vi "ECG.vi"() -> ()   [LabVIEW 2016]
uses:
  <vilib>/Analysis/3filter.llb/Filter Passband Type.ctl
  <vilib>/ptbypt/NI_PtbyPt.lvlib
  <vilib>/Analysis/NI_AALBase.lvlib
panel:
  in  "stop 2":bool
  in  "stop":bool
  in  "submit":bool
  out "Prompt":string="Update or Confirm the Following Information:"
  out "Pat":string="Patient Name:"
  out "Dat":string="Date/Time:"
  out "time string 2":string
  out "date string 2":string
  in  "Name 2":string="Doe, John"
  in  "Notes:":string
  out "Box":string
  in  "Notes:":string
  out "String":string
  out "Elapsed Time (s)":dbl format="%<%H:%M:%S>t"
  out "time string":string
  out "date string":string
  out "Heart":bool
  in  "Name":string="Doe, John"
  in  "T Thresh":string="100"
  in  "B Thresh":string="60"
  out "Bradycardia":bool
  out "Tachycardia":bool
  out "HR":dbl=56.0
  out "String 2":string
  out "Waveform Chart":dbl(graph)
  # "Patient Name:"
  # "Date/Time:"
  # "HR"
  # "bpm"
  # "Set Thresholds:"
  # "Bradycardia"
  # "Tachycardia"
  # "Time Elapsed:"
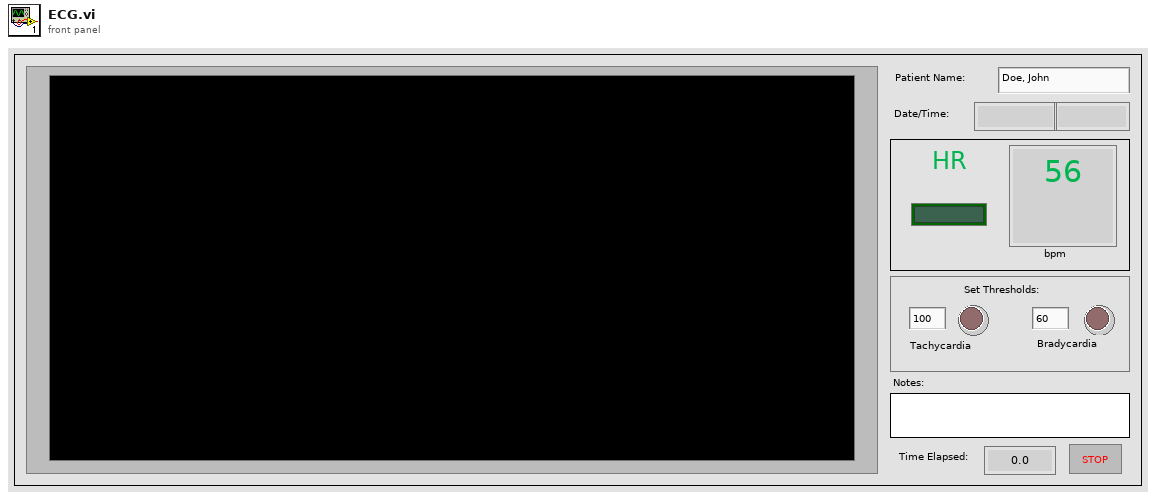
[diagram p1: front panel]
types:
  T1 = typedef "NI_AALBase.lvlib/Filter Passband Type.ctl" = enum32{"Lowpass", "Highpass", "Bandpass", "Bandstop"}
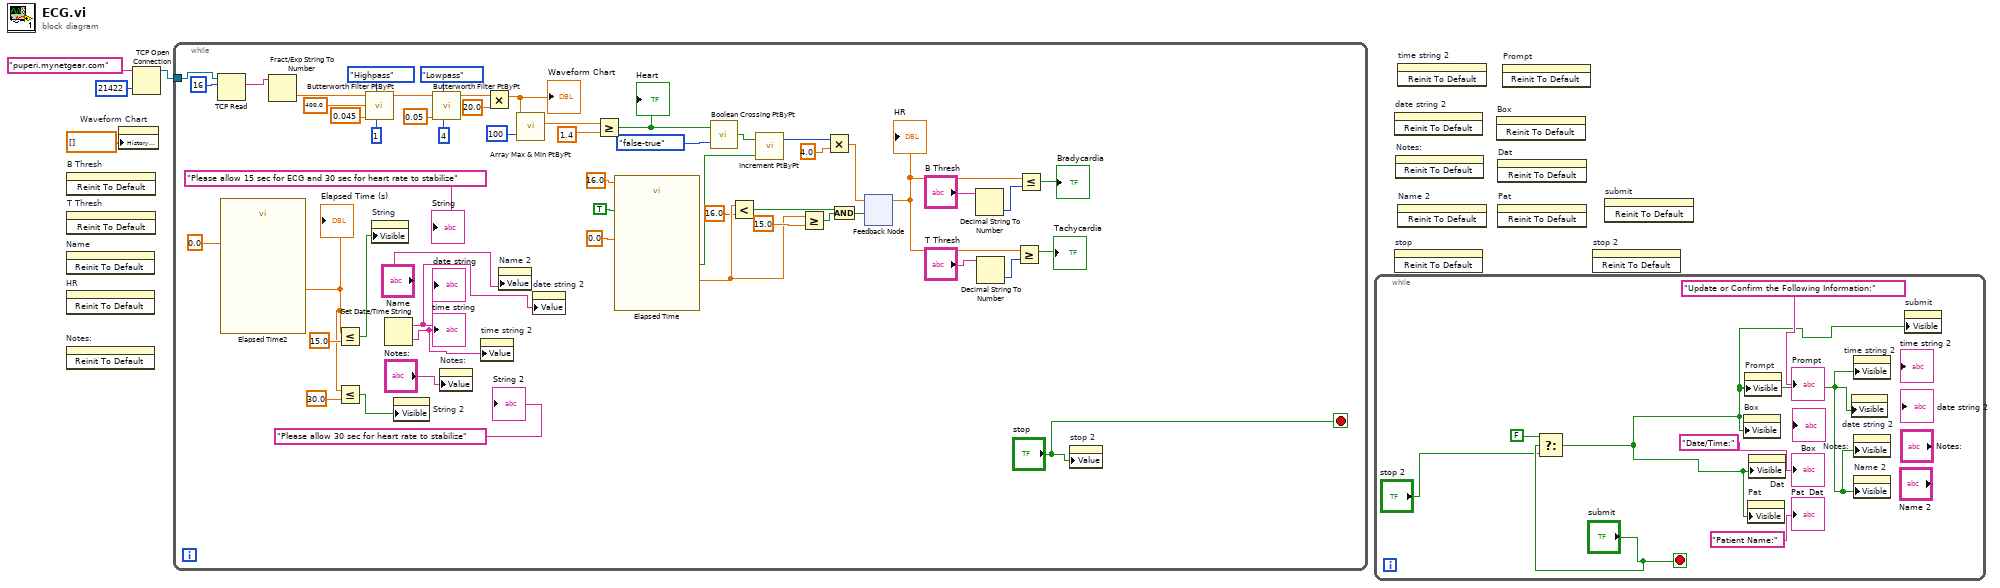
[diagram p0: block diagram]
diagram:
  n1 = invoke on="Name" class="Str" method="Reinit To Default"() -> ()  [unwired: 3 in, 3 out]
  n2 = invoke on="HR" class="DigNum (strict)" method="Reinit To Default"() -> ()  [unwired: 3 in, 3 out]
  n3 = invoke on="Notes:" class="Str" method="Reinit To Default"() -> ()  [unwired: 3 in, 3 out]
  n4 = invoke on="B Thresh" class="Str" method="Reinit To Default"() -> ()  [unwired: 3 in, 3 out]
  n5 = invoke on="T Thresh" class="Str" method="Reinit To Default"() -> ()  [unwired: 3 in, 3 out]
  n6 = property on="Waveform Chart" class="WFChart (strict)"("History Data"=dbl[] []) -> ()  [unwired: 2 in, 2 out]
  n7 = TCP Open Connection(address="puperi.mynetgear.com", remote port or service name=u16 21422) -> (connection ID=w2:refnum<k5>)  [unwired: 3 in, 1 out]
  n8 = while {
    tunnel: w2 -> [w58]
    stop <- "stop" stop-if-true
    n9 = TCP Read(connection ID=w58, bytes to read=16) -> (data out=w51:string)  [unwired: 3 in, 2 out]
    n10 = call "Elapsed Time2"("Set Start Time (s)"=0.0) -> ("Elapsed Time (s)"=w8:dbl)  [unwired: 11 in, 7 out]
    "Elapsed Time (s)" <- w8
    n11 = Fract/Exp String To Number(string=w51) -> (number=w53:dbl)  [unwired: 3 in, 1 out]
    n12 = Less Or Equal?(x=w8, y=15.0) -> (x <= y?=w14:bool)
    n13 = Less Or Equal?(x=w8, y=30.0) -> (x <= y?=w5:bool)
    n14 = call <vilib>:"Butterworth Filter PtByPt.vi"("order"=1, "filter type"=Filter_Passband_Type."Highpass", "low cutoff freq: fl"=0.045, "sampling freq: fs"=400.0, "x"=w53) -> ("Filtered x"=w27:dbl)  [unwired: 4 in, 1 out]
    n15 = property on="String" class="Str"("Visible"=w14) -> ()  [unwired: 2 in, 2 out]
    n16 = Get Date/Time String() -> (date string=w10:string, time string=w11:string)  [unwired: 3 in]
    "date string" <- w10
    "time string" <- w11
    n17 = property on="String 2" class="Str"("Visible"=w5) -> ()  [unwired: 2 in, 2 out]
    n18 = call <vilib>:"Butterworth Filter PtByPt.vi"("order"=4, "filter type"=Filter_Passband_Type."Lowpass", "low cutoff freq: fl"=0.05, "x"=w27) -> ("Filtered x"=w22:dbl)  [unwired: 5 in, 1 out]
    n19 = property on="Notes:" class="Str"("Value"="Notes:") -> ()  [unwired: 2 in, 2 out]
    n20 = property on="time string 2" class="Str"("Value"=w11) -> ()  [unwired: 2 in, 2 out]
    n21 = Multiply(x=w22, y=20.0) -> (x*y=w18:dbl)
    "Waveform Chart" <- w18
    n22 = property on="Name 2" class="Str"("Value"="Name") -> ()  [unwired: 2 in, 2 out]
    n23 = call <vilib>:"Array Max & Min PtByPt.vi"("input data point"=w18, "sample length"=100) -> ("max value"=w21:dbl)  [unwired: 1 in, 4 out]
    n24 = property on="date string 2" class="Str"("Value"=w10) -> ()  [unwired: 2 in, 2 out]
    n25 = Greater Or Equal?(x=w21, y=1.4) -> (x >= y?=w17:bool)
    "Heart" <- w17
    n26 = call "Elapsed Time"("Time Target (s)"=16.0, "Auto Reset"=TRUE, "Set Start Time (s)"=0.0) -> ("Elapsed Time (s)"=w40:dbl, "Time has Elapsed"=w29:bool)  [unwired: 9 in, 6 out]
    n27 = call <vilib>:"Boolean Crossing PtByPt.vi"("direction"=enum16{"either", "false-true", "true-false"}."false-true", "input"=w17) -> ("crossing"=w20:bool)  [unwired: 1 in]
    n28 = Less?(x=w40, y=16.0) -> (x < y?=w39:bool)
    n29 = call <vilib>:"Increment PtByPt.vi"("initialize"=w29, "activate"=w20) -> ("counter"=w23:u32)  [unwired: 1 out]
    n30 = Greater Or Equal?(x=w40, y=15.0) -> (x >= y?=w41:bool)
    n31 = Multiply(x=w23, y=4.0) -> (x*y=w43:dbl)
    n32 = And(x=w39, y=w41) -> (x .and. y?=w38:bool)
    n33 = feedback-in #1(w43, w38) -> ()
    n34 = feedback #1() -> (w36:dbl)  [unwired: 1 in]
    "HR" <- w36
    n35 = Decimal String To Number(string="B Thresh") -> (number=w30:i32)  [unwired: 2 in, 1 out]
    n36 = Decimal String To Number(string="T Thresh") -> (number=w31:i32)  [unwired: 2 in, 1 out]
    n37 = Greater Or Equal?(x=w36, y=w31) -> (x >= y?=→"Tachycardia":bool)
    n38 = Less Or Equal?(x=w36, y=w30) -> (x <= y?=→"Bradycardia":bool)
    n39 = property on="stop 2" class="Bool (strict)"("Value"="stop") -> ()  [unwired: 2 in, 2 out]
    "String" <- "Please allow 15 sec for ECG and 30 sec for heart rate to stabilize"
    "String 2" <- "Please allow 30 sec for heart rate to stabilize"
  }
  n40 = while {
    stop <- "submit" stop-if-true
    n41 = Select(t=FALSE, s="submit", f="stop 2") -> (s? t:f=w61:bool)
    n42 = property on="Box" class="Str"("Visible"=w61) -> ()  [unwired: 2 in, 2 out]
    n43 = property on="Prompt" class="Str"("Visible"=w61) -> ()  [unwired: 2 in, 2 out]
    n44 = property on="Pat" class="Str"("Visible"=w61) -> ()  [unwired: 2 in, 2 out]
    n45 = property on="Dat" class="Str"("Visible"=w61) -> ()  [unwired: 2 in, 2 out]
    n46 = property on="date string 2" class="Str"("Visible"=w61) -> ()  [unwired: 2 in, 2 out]
    n47 = property on="time string 2" class="Str"("Visible"=w61) -> ()  [unwired: 2 in, 2 out]
    n48 = property on="Notes:" class="Str"("Visible"=w61) -> ()  [unwired: 2 in, 2 out]
    n49 = property on="Name 2" class="Str"("Visible"=w61) -> ()  [unwired: 2 in, 2 out]
    n50 = property on="submit" class="Bool"("Visible"=w61) -> ()  [unwired: 2 in, 2 out]
    "Dat" <- "Date/Time:" ("Dat")
    "Pat" <- "Patient Name:" ("Pat")
    "Prompt" <- "Update or Confirm the Following Information:" ("Prompt")
  }
  n51 = invoke on="date string 2" class="Str" method="Reinit To Default"() -> ()  [unwired: 3 in, 3 out]
  n52 = invoke on="stop" class="Bool (strict)" method="Reinit To Default"() -> ()  [unwired: 3 in, 3 out]
  n53 = invoke on="Notes:" class="Str" method="Reinit To Default"() -> ()  [unwired: 3 in, 3 out]
  n54 = invoke on="time string 2" class="Str" method="Reinit To Default"() -> ()  [unwired: 3 in, 3 out]
  n55 = invoke on="Name 2" class="Str" method="Reinit To Default"() -> ()  [unwired: 3 in, 3 out]
  n56 = invoke on="Box" class="Str" method="Reinit To Default"() -> ()  [unwired: 3 in, 3 out]
  n57 = invoke on="Dat" class="Str" method="Reinit To Default"() -> ()  [unwired: 3 in, 3 out]
  n58 = invoke on="Pat" class="Str" method="Reinit To Default"() -> ()  [unwired: 3 in, 3 out]
  n59 = invoke on="Prompt" class="Str" method="Reinit To Default"() -> ()  [unwired: 3 in, 3 out]
  n60 = invoke on="stop 2" class="Bool (strict)" method="Reinit To Default"() -> ()  [unwired: 3 in, 3 out]
  n61 = invoke on="submit" class="Bool" method="Reinit To Default"() -> ()  [unwired: 3 in, 3 out]
